vi "split query string.vi"(10 "delimiter":string="&", 11 "query":string) -> (3 "query values":cluster{"key":string, "value":string}[](array[cluster]))   [LabVIEW 2013, in "uniform resource locator.lvlib"]
uses:
  uniform resource locator.lvlib
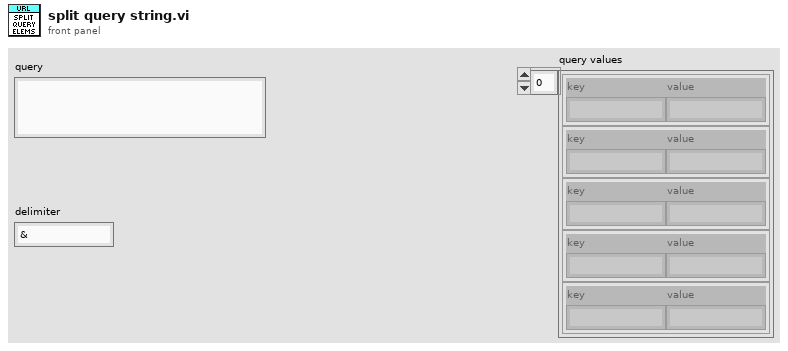
[diagram p1: front panel]
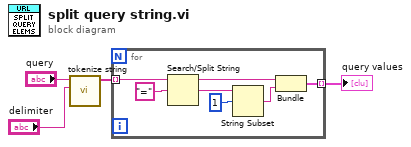
[diagram p0: block diagram]
diagram:
  n1 = call "tokenize string.vi"("delimiter"="delimiter", "raw path"="query") -> ("segments"=w2:string[])  [unwired: 9 in]
  n2 = for {
    tunnel: w2 -> [w11] mode=indexing
    tunnel: [w5] -> w1 mode=indexing
    n3 = Search/Split String(string=w11, search string/char (-)="=") -> (substring before match=w6:string, match + rest of string=w9:string)  [unwired: 1 in, 1 out]
    n4 = String Subset(string=w9, offset (0)=1) -> (substring=w7:string)  [unwired: 1 in]
    n5 = Bundle("String"=w6, "String"=w7) -> (w5:cluster{"String":string, "String":string})  [unwired: 1 in]
  }
  "query values" <- w1
